vi "Take Composite Image.vi"(4 "Interrupt Reference":refnum<vi>, 6 "Slider Reference":refnum<vi>, 7 "Quality":enum16{"perfect", "high", "medium", "low"}(ring), 8 "error in (no error)":errorcluster, 9 "Image Name":string="composite image", 10 "Points":refnum<class "Vec3d.lvclass">[](array[class]), 11 "Gantry in":refnum<class "Gantry.lvclass">) -> (0 "error out":errorcluster, 2 "Physical Image":T1, 3 "Gantry out":refnum<class "Gantry.lvclass">)   [LabVIEW 2024, in "Gantry.lvclass"]
uses:
  Gantry.lvclass
  Utils/Type Definitions/Physical Image.ctl
  Vec3d Class/Vec3d.lvclass
  <vilib>/vision/Image Controls.llb/IMAQ Image.ctl
  FlexWorktable/FlexWorktable.lvclass
  Gantry.lvclass/Gantry.ctl
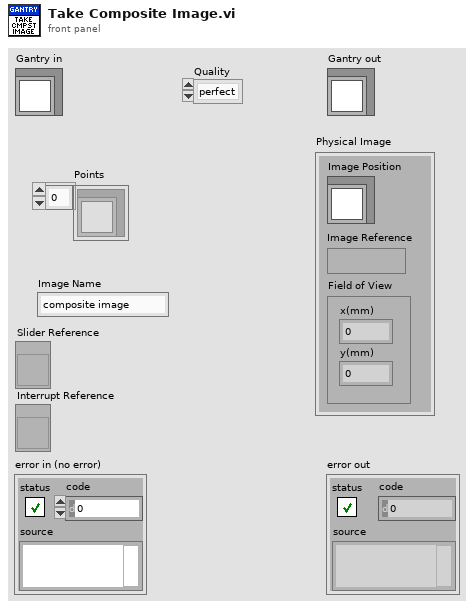
[diagram p1: front panel]
types:
  T1 = typedef "Physical Image.ctl" = cluster{"Image Position":refnum<class "Vec3d.lvclass">, "Image Reference":T2, "Field of View":cluster{"x(mm)":dbl, "y(mm)":dbl}}
  T2 = typedef "IMAQ Image.ctl" = refnum<image>
  T3 = typedef "FlexWorktable.lvclass/Camera State.ctl" = cluster{"Group":i32, "Open?":bool, "Driver":T4, "serial number":string, "Field of View":cluster{"x-mm":dbl, "y-mm":dbl}, "Rotation":T5, "Vertical Mirror":bool}
  T4 = typedef "Vision.lvlib/camera driver.ctl" = enum16{"none", "wmf", "imaqdx", "peak"}
  T5 = typedef "Camera Rotation.ctl" = enum16{"0", "90", "180", "270"}
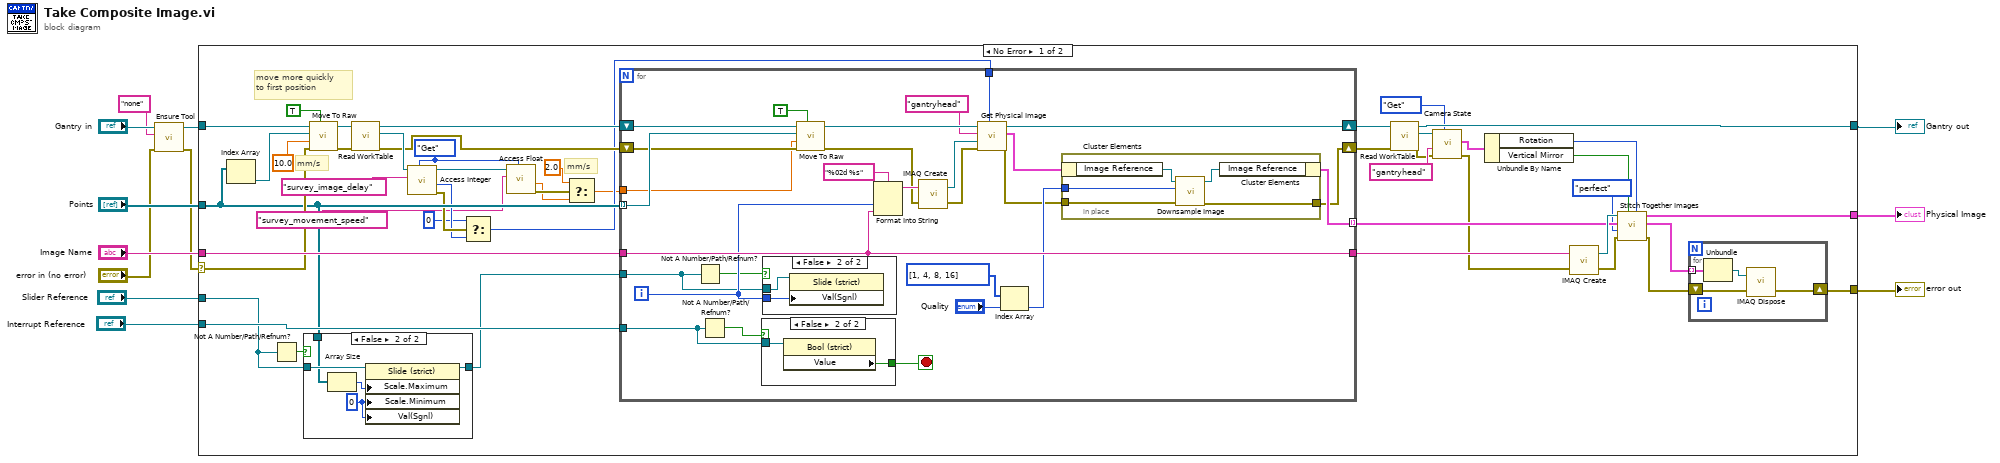
[diagram p0: block diagram]
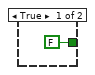
[diagram p3: hidden frame]
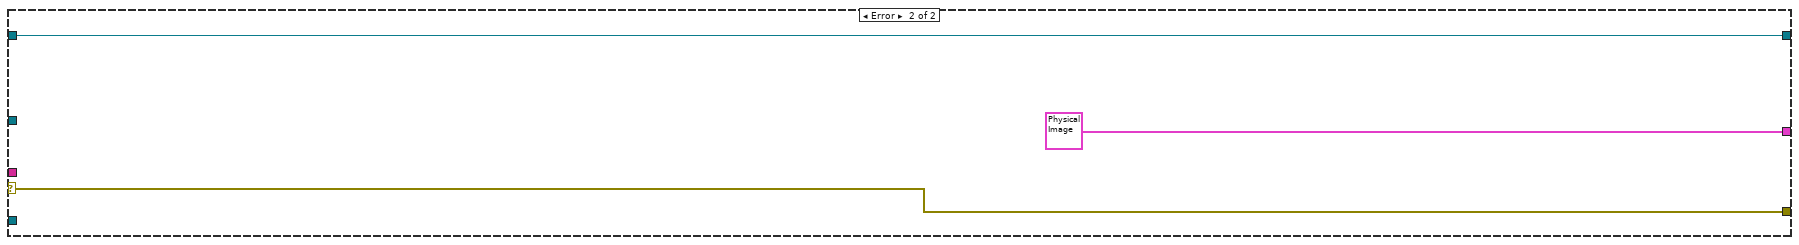
[diagram p5: hidden frame]
diagram:
  n1 = call "Ensure Tool.vi"("error in (no error)"="error in (no error)", "Tool Name"="none", "Gantry in"="Gantry in") -> ("error out"=w4:errorcluster, "Gantry out"=w6:refnum<class "Gantry.lvclass">)  [unwired: 7 in]
  n2 = case shown="No Error" w4 {
    selector: w4 -> [w47 w111]
    tunnel: [w52 w111] -> w10
    tunnel: [w21 w110] -> w8
    tunnel: w6 -> [w49 w110]
    tunnel: "Points" -> [w44 _]
    tunnel: "Image Name" -> [w58 _]
    tunnel: [w55 T1 {"Image Position"=refnum, "Image Reference"=refnum, "Field of View"={"x(mm)"=0.0, "y(mm)"=0.0}} ("Composite Physical Image")] -> w9
    tunnel: "Slider Reference" -> [w43 _]
    tunnel: "Interrupt Reference" -> [w46 _]
    frame No Error {
      w35 = enum16{"Get", "Set"}."Get" ("Get/Set")
      # "mm/s"
      # "move more quickly\nto first position"
      # "mm/s"
      n3 = Index Array(array=w44) -> (element=w48:refnum<class "Vec3d.lvclass">)  [unwired: 1 in]
      n4 = Not A Number/Path/Refnum?(number/path/refnum=w43) -> (NaN/Path/Refnum?=w45:bool)
      n5 = case shown="False" w45 {
        tunnel: w43 -> [w61 w66]
        tunnel: w44 -> [_ w64]
        tunnel: [w61 w63] -> w42
        frame True {
        }
        frame False {
          w62 = u8 0 ("Value (Signaling)")
          n6 = Array Size(array=w64) -> (size(s)=w65:i32)
          n7 = property on="Property Node" class="Slide (strict)"(reference=w66, "Scale.Maximum"=w65, "Scale.Minimum"=w62, "Val(Sgnl)"=w62) -> (reference out=w63:refnum<vi>)  [unwired: 1 in, 1 out]
        }
      }
      n8 = call-dynamic "Move To Raw.vi"("Wait?"=TRUE, "error in"=w47, "Speed"=10.0, "Destination"=w48, "Gantry in"=w49) -> ("error out"=w39:errorcluster, "Gantry out"=w40:refnum<class "Gantry.lvclass">)  [unwired: 5 in]
      n9 = call-dynamic "Read WorkTable.vi"("error in"=w39, "Gantry Class in"=w40) -> ("error out"=w34:errorcluster, "Worktable"=w37:refnum<class "FlexWorktable.lvclass">, "Gantry Class out"=w38:refnum<class "Gantry.lvclass">)  [unwired: 7 in]
      n10 = call-dynamic "Access Integer.vi"("Get/Set"=w35, "Key"="survey_image_delay", "FlexWorktable in"=w37) -> ("error out"=w32:errorcluster, "Value out"=w31:i32, "FlexWorktable out"=w36:refnum<class "FlexWorktable.lvclass">)  [unwired: 6 in]
      n11 = Select(t=0, s=w32, f=w31) -> (s? t:f=w29:i32)
      n12 = call-dynamic "Access Float.vi"("Get/Set"=w35, "Key"="survey_movement_speed", "FlexWorktable in"=w36) -> ("error out"=w27:errorcluster, "Value out"=w25:dbl)  [unwired: 6 in, 1 out]
      n13 = Select(t=2.0, s=w27, f=w25) -> (s? t:f=w24:dbl)
      n14 = for {
        shift-right: [w73] -> w17
        shift-left: w34 -> [w88]
        shift-right: [w96] -> w23
        shift-left: w38 -> [w98]
        tunnel: w44 -> [w94] mode=indexing
        tunnel: [w75] -> w59 mode=indexing
        tunnel: [w87] -> w57
        tunnel: w58 -> [w87]
        tunnel: w42 -> [w83]
        tunnel: w46 -> [w81]
        tunnel: w29 -> [w72]
        tunnel: w24 -> [w71]
        i -> [w85]
        stop <- w80 stop-if-true
        n15 = Not A Number/Path/Refnum?(number/path/refnum=w83) -> (NaN/Path/Refnum?=w84:bool)
        n16 = Not A Number/Path/Refnum?(number/path/refnum=w81) -> (NaN/Path/Refnum?=w82:bool)
        n17 = case shown="False" w82 {
          tunnel: w81 -> [_ w106]
          tunnel: [FALSE ("Value") w105] -> w80
          frame True {
          }
          frame False {
            n18 = property on="Property Node" class="Bool (strict)"(reference=w106) -> ("Value"=w105:bool)  [unwired: 1 in, 2 out]
          }
        }
        n19 = case shown="False" w84 {
          tunnel: w85 -> [_ w108]
          tunnel: w83 -> [_ w107]
          frame True {
          }
          frame False {
            n20 = property on="Property Node" class="Slide (strict)"(reference=w107, "Val(Sgnl)"=w108) -> ()  [unwired: 1 in, 2 out]
          }
        }
        n21 = call-dynamic "Move To Raw.vi"("Wait?"=TRUE, "error in"=w88, "Speed"=w71, "Destination"=w94, "Gantry in"=w98) -> ("error out"=w91:errorcluster, "Gantry out"=w97:refnum<class "Gantry.lvclass">)  [unwired: 5 in]
        n22 = Format Into String(format string="%02d %s", w85, w87) -> (resulting string=w92:string)  [unwired: 2 in, 1 out]
        n23 = call "IMAQ Create"("Image Name"=w92, "error in (no error)"=w91) -> ("New Image"=w89:T2, "error out"=w90:errorcluster)  [unwired: 3 in]
        n24 = call-dynamic "Get Physical Image.vi"("Delay(milliseconds)"=w72, "error in"=w90, "Image In"=w89, "Camera Name"="gantryhead", "Gantry in"=w97) -> ("error out"=w74:errorcluster, "Physical Image"=w76:T1, "Gantry out"=w96:refnum<class "Gantry.lvclass">)  [unwired: 4 in]
        n25 = Index Array(array=i32[] [1, 4, 8, 16], index="Quality") -> (element=w77:i32)
        n26 = in-place {
          in-place-border: w77 -> [w103]
          in-place-border: w74 -> [w100]
          in-place-border: [w99] -> w73
          n27 = in-place-cluster #1(w76) -> ("Image Reference"=w102:T2)
          n28 = call "Downsample Image.vi"("error in"=w100, "Reduction Factor"=w103, "Refnum in"=w102) -> ("error out"=w99:errorcluster, "Refnum out"=w101:T2)  [unwired: 7 in]
          n29 = in-place-cluster #1("Image Reference"=w101) -> (w75:T1)
        }
      }
      n30 = call-dynamic "Read WorkTable.vi"("error in"=w17, "Gantry Class in"=w23) -> ("error out"=w16:errorcluster, "Worktable"=w22:refnum<class "FlexWorktable.lvclass">, "Gantry Class out"=w21:refnum<class "Gantry.lvclass">)  [unwired: 7 in]
      n31 = call-dynamic "Camera State.vi"("Get/Set"=enum16{"Get", "Set"}."Get", "error in (no error)"=w16, "Camera Name"="gantryhead", "FlexWorktable in"=w22) -> ("error out"=w15:errorcluster, "State"=w18:T3)  [unwired: 5 in, 1 out]
      n32 = Unbundle By Name(w18) -> ("Rotation"=w13:T5, "Vertical Mirror"=w14:bool)
      n33 = call "IMAQ Create"("Image Name"=w57, "error in (no error)"=w15) -> ("New Image"=w60:T2, "error out"=w56:errorcluster)  [unwired: 3 in]
      n34 = call "Stitch Together Images.vi"("Rotation"=w13, "Vertical Mirror"=w14, "error in"=w56, "Quality"=enum16{"perfect", "high", "medium", "low"}."perfect", "Physical Images in"=w59, "Image Dst"=w60) -> ("error out"=w53:errorcluster, "Physical Images out"=w54:T1[], "Composite Physical Image"=w55:T1)  [unwired: 3 in]
      n35 = for {
        tunnel: w54 -> [w70] mode=indexing
        shift-right: [w67] -> w52
        shift-left: w53 -> [w68]
        n36 = Unbundle(w70) -> ("Image Reference"=w69:T2)  [unwired: 2 out]
        n37 = call "IMAQ Dispose"("Image"=w69, "error in (no error)"=w68) -> ("error out"=w67:errorcluster)  [unwired: 4 in]
      }
    }
    frame Error {
    }
  }
  "error out" <- w10
  "Gantry out" <- w8
  "Physical Image" <- w9
